vi "Popup.vi"(0 "Back":bool) -> ()   [LabVIEW 2023]
doc: "This is Popup VI, which pops-up when the main VI makes it pop-up."
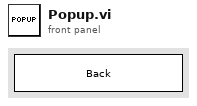
[diagram p1: front panel]
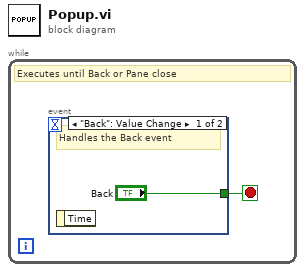
[diagram p0: block diagram]
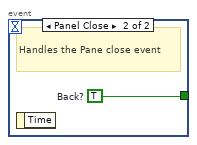
[diagram p2: hidden frame]
diagram:
  n1 = while {
    stop <- w1 stop-if-true
    # "Executes until Back or Pane close"
    n2 = event shown="[0] \"Back\": Value Change" {
      selector: _ -> [_ _]
      dyn-events: _ -> [_ _]
      timeout: _ -> [_ _]
      tunnel: ["Back" w3] -> w1
      event "Back": Value Change {
        # "Handles the Back event"
        n3 = event-data() -> ()  [unwired: 1 in, 1 out]
      }
      event Panel Close {
        w3 = TRUE  # Back?
        # "Handles the Pane close event"
        n4 = event-data() -> ()  [unwired: 1 in, 1 out]
      }
    }
  }
